vi "Kalibrationsprogramm dodenhoeft.vi"(2 "Delay [ms]":u32=10000, 3 "Messzeit [ms]":u32=7000, 4 "B-Feld":dbl=4.0, 5 "error in (no error)":errorcluster, 6 "Startwert (V)":dbl=-6.0 min=-30.0 max=30.0 step=0.01, 7 "Stepsize (V)":dbl=1.0 min=0.0, 8 "Endwert (V)":dbl=6.0 min=-30.0 max=30.0 step=0.01) -> (15 "Ausgabe-Cluster":T1={" I (A)"=-6.000000000000021, "Voltage"=0.143902, "B-Feld"=4.0, "Timestamp"=3443775799.1979947} {"Timestamp" format="%#_6f"}, 19 "error out":errorcluster)   [LabVIEW 2009]
uses:
  Instance           2 16Saved   Yokogawa .vi
  <vilib>/Utility/file.llb/Write To Spreadsheet File (DBL).vi
panel:
  out "XY Graph":cluster{dbl[], dbl[]}(graph)={[-6.000000000000005, -4.990000000000027, -3.9901000000000244, -2.9900990000000083, -1.9999999999999865, -0.9900000000000079, 2.400857290751901e-15, 1.000000000000001, 2.0000000000000018, 3.0099999999999802, 4.009899999999982, 5.009900999999998, 6.00000000000002, 4.990000000000042, 3.9901000000000395, 2.999999999999979, 1.9900000000000007, 0.9999999999999987, -1.5439038936193583e-15, -1.0000000000000018, -2.0000000000000027, -3.009999999999981, -4.009899999999983, -5.009900999999999, -6.000000000000021], [0.1439003448275862, 0.14384071428571427, 0.14379167857142858, 0.14374593103448274, 0.14371203448275863, 0.14368321428571423, 0.1436658620689656, 0.1436561034482759, 0.14365485714285722, 0.14366034482758627, 0.14367178571428574, 0.1436978571428571, 0.14372814285714283, 0.14369535714285714, 0.1436752857142857, 0.14366071428571434, 0.14365396428571436, 0.14365448275862072, 0.14366448275862076, 0.14368586206896547, 0.1437107142857143, 0.14374785714285715, 0.14379375862068966, 0.1438423214285714, 0.1439047142857143]}
  in  "file path (dialog if empty)":path=path "D:/UserData/Matthias/Messungen/MgOZnO/130215/130215_259a_kalib4T_1.txt"
  out "Done":bool=TRUE
  out "Data":bool
  out "UI":dbl=-6.000000000000021
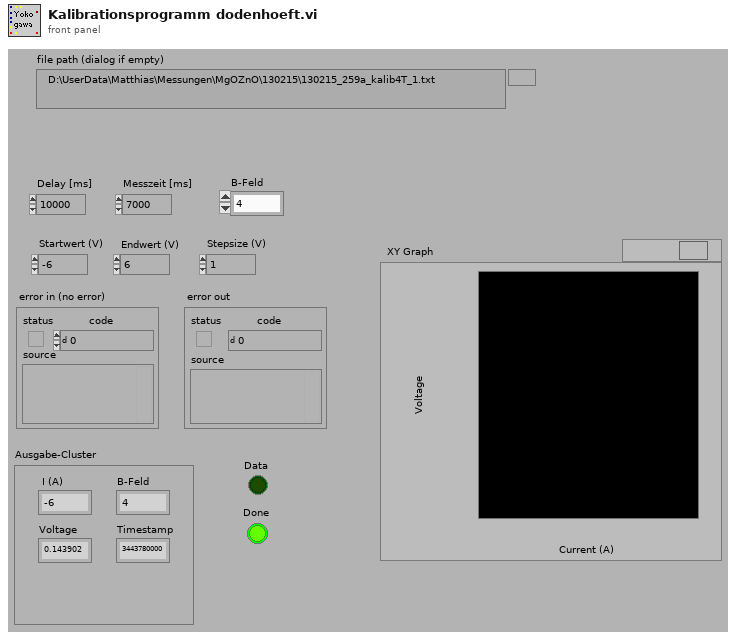
[diagram p1: front panel]
types:
  T1 = cluster{" I (A)":dbl, "Voltage":dbl, "B-Feld":dbl, "Timestamp":dbl}
  T2 = cluster{"UI":dbl, "capacitance":dbl, "B-Feld":dbl, dbl}
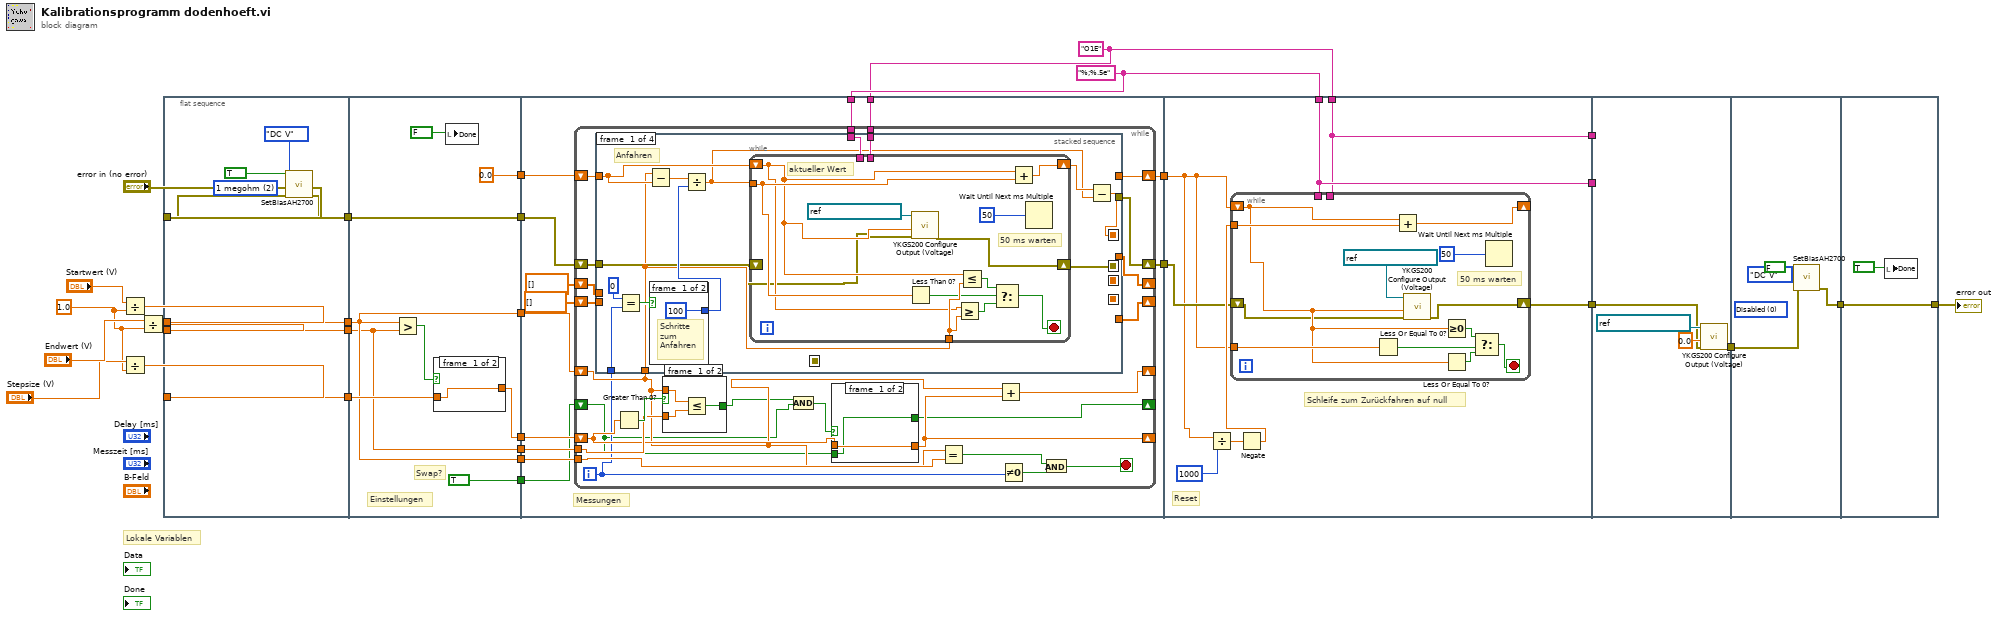
[diagram p0: block diagram]
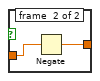
[diagram p2: hidden frame]
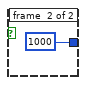
[diagram p3: hidden frame]
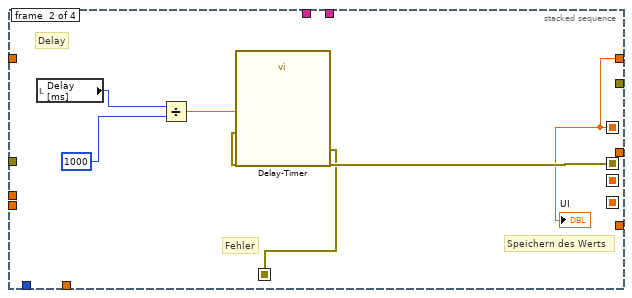
[diagram p4: hidden frame]
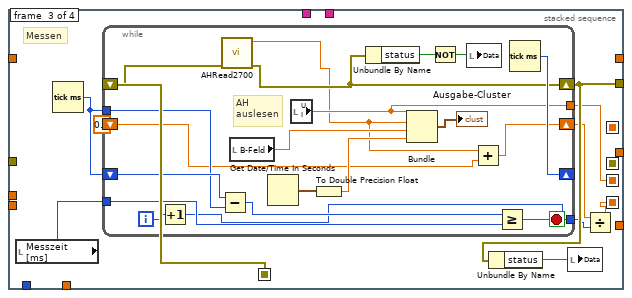
[diagram p5: hidden frame]
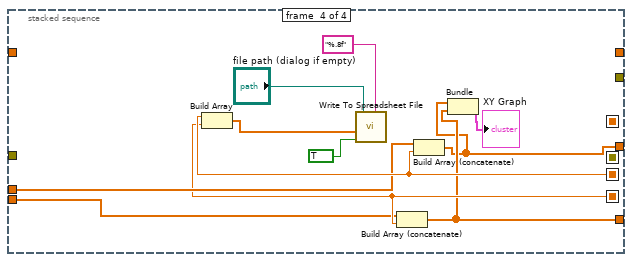
[diagram p6: hidden frame]
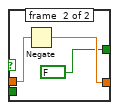
[diagram p7: hidden frame]
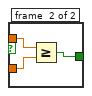
[diagram p8: hidden frame]
diagram:
  w7 = 1.0 ("y")
  w19 = "O1E"
  w20 = "%;%.5e"
  # "Lokale Variablen"
  n1 = Divide(x="Startwert (V)", y=w7) -> (x/y=w12:dbl)
  n2 = Divide(x="Stepsize (V)", y=w7) -> (x/y=w8:dbl)
  n3 = Divide(x="Endwert (V)", y=w7) -> (x/y=w10:dbl)
  n4 = flat-sequence {
    tunnel: "error in (no error)" -> [w33]
    tunnel: w8 -> [w35]
    tunnel: w10 -> [w36]
    tunnel: w12 -> [w37]
    tunnel: [w37] -> w6
    tunnel: [w36] -> w5
    tunnel: [w35] -> w4
    tunnel: [w32] -> w3
    tunnel: [w43] -> w29
    tunnel: [w44] -> w28
    tunnel: [w43] -> w27
    tunnel: [w42] -> w26
    tunnel: [0.0] -> w25
    tunnel: [w38] -> w24
    tunnel: [TRUE] -> w23
    tunnel: w6 -> [w43]
    tunnel: w5 -> [w42]
    tunnel: w4 -> [w45]
    tunnel: w3 -> [w38]
    tunnel: w29 -> [w62]
    tunnel: w28 -> [w60]
    tunnel: w27 -> [w61]
    tunnel: w26 -> [w59]
    tunnel: w25 -> [w58]
    tunnel: w20 -> [w57]
    tunnel: w19 -> [w56]
    tunnel: w24 -> [w55]
    tunnel: w23 -> [w53]
    tunnel: [w54] -> w22
    tunnel: [w52] -> w21
    tunnel: w22 -> [w178]
    tunnel: w21 -> [w176]
    tunnel: w20 -> [w175]
    tunnel: w19 -> [w174]
    tunnel: [w177] -> w17
    tunnel: [w175] -> w15
    tunnel: [w174] -> w14
    tunnel: w17 -> [w195]
    tunnel: w15 -> [_]
    tunnel: w14 -> [_]
    tunnel: [w194] -> w1
    tunnel: [w201] -> w2
    tunnel: w1 -> [w198]
    tunnel: [w203] -> w18
    tunnel: w2 -> [w203]
    frame #0 {
      w30 = 2 items=["Disabled", "100 megohm", "1 megohm"] ("Bias (Off)")
      n5 = call "SetBiasAH2700.vi"("error in (no error)"=w33, "Bias (Off)"=w30, "V/A ?"=enum16{"DC V", "DC A"}."DC V", "On/Off"=TRUE) -> ("error out"=w32:errorcluster)  [unwired: 7 in]
    }
    frame #1 {
      # "Einstellungen"
      # "Swap?"
      n6 = Greater?(x=w43, y=w42) -> (0:w46:bool)
      n7 = case shown="False" w46 {
        tunnel: w45 -> [w47 w49]
        tunnel: [w47 w48] -> w44
        frame #0 {
        }
        frame #1 {
          n8 = Negate(x=w49) -> (-x=w48:dbl)
        }
      }
      n9 = local write "Done"(FALSE) -> ()
    }
    frame #2 {
      # "Messungen"
      n10 = while {
        shift-right: [w76] -> _
        shift-left: w62 -> [w78]
        tunnel: w61 -> [w87]
        shift-right: [w77] -> _
        shift-left: w60 -> [w84]
        tunnel: w59 -> [w85]
        shift-right: [w79] -> w52
        shift-left: w58 -> [w83]
        tunnel: w57 -> [w82]
        tunnel: w56 -> [w81]
        shift-right: [w75] -> w54
        shift-left: w55 -> [w80]
        shift-right: [w70] -> _
        shift-left: w53 -> [w68]
        shift-right: [w65] -> _
        shift-left: dbl[] [] -> [w66]
        shift-right: [w64] -> _
        shift-left: dbl[] [] -> [w63]
        i -> [w74]
        stop <- w71 stop-if-true
        n11 = stacked-sequence {
          seq-local: [w93 _ _ _] -> [_ w121 _ _]
          seq-local: [_ w120 _ _] -> [_ _ w129 _]
          seq-local: [w88 _ _ _] -> [_ w116 _ _]
          seq-local: [_ _ w125 _] -> [_ _ _ w158]
          seq-local: [_ _ w122 _] -> [_ _ _ w156]
          tunnel: w74 -> [w100 _ _ _]
          tunnel: w83 -> [w92 _ _ _]
          tunnel: w78 -> [w91 _ _ _]
          tunnel: w82 -> [w96 _ _ _]
          tunnel: w81 -> [w95 _ _ _]
          tunnel: w80 -> [w94 _ _ _]
          tunnel: [_ w116 _ _] -> w79
          tunnel: [_ _ w128 _] -> w75
          tunnel: w66 -> [_ _ _ w157]
          tunnel: [_ _ _ w153] -> w65
          tunnel: [_ _ _ w154] -> w64
          tunnel: w63 -> [_ _ _ w155]
          frame #0 {
            # "Anfahren"
            n12 = Equal?(x=0, y=w100) -> (x = y?=w101:bool)
            n13 = Subtract(x=w91, y=w92) -> (x-y=w98:dbl)
            n14 = case shown="True" w101 {
              tunnel: [100 1000] -> w97
              frame #0 {
                # "Schritte\nzum\nAnfahren"
              }
              frame #1 {
              }
            }
            n15 = Divide(x=w98, y=w97) -> (x/y=w89:dbl)
            n16 = while {
              shift-right: [w113] -> w90
              shift-left: w92 -> [w105]
              tunnel: w91 -> [w110]
              tunnel: w89 -> [w111]
              tunnel: w96 -> [_]
              tunnel: w95 -> [_]
              shift-right: [w102] -> w93
              shift-left: w94 -> [w104]
              stop <- w106 stop-if-true
              # "50 ms warten"
              # "aktueller Wert"
              n17 = Less Than 0?(x=w111) -> (x < 0?=w109:bool)
              n18 = call <instrlib>:"YKGS200 Configure Output (Voltage).vi"("error in (no error)"=w104, "Voltage Level (0.0 V)"=w105, "VISA resource name"=refnum<visa-resource-name> "GPIB0::6::INSTR") -> ("error out"=w102:errorcluster)  [unwired: 7 in, 1 out]
              n19 = Greater Or Equal?(x=w105, y=w110) -> (x >= y?=w107:bool)
              n20 = Less Or Equal?(x=w105, y=w110) -> (x <= y?=w108:bool)
              n21 = Select(t=w108, s=w109, f=w107) -> (s? t:f=w106:bool)
              n22 = Add(x=w105, y=w111) -> (x+y=w113:dbl)
              n23 = Wait Until Next ms Multiple(millisecond multiple=50) -> ()  [unwired: 1 out]
            }
            n24 = Subtract(x=w90, y=w89) -> (x-y=w88:dbl)
          }
          frame #1 {
            # "Delay"
            # "Speichern des Werts"
            # "Fehler"
            n25 = local read "Delay [ms]"() -> (w117:u32)
            n26 = Divide(x=w117, y=u32 1000) -> (x/y=w118:dbl)
            n27 = call "Delay-Timer"("error in (no error)"=w121, "Delay Time (s)"=w118) -> ("error out"=w120:errorcluster)  [unwired: 9 in]
            "UI" <- w116
          }
          frame #2 {
            # "Messen"
            n28 = local read "Messzeit [ms]"() -> (w130:u32)
            n29 = Tick Count (ms)() -> (millisecond timer value=w131:u32)
            n30 = while {
              shift-right: [w151] -> _
              shift-left: w131 -> [w150]
              tunnel: w131 -> [w149]
              tunnel: w130 -> [w147]
              shift-right: [w133] -> w128
              shift-left: w129 -> [w134]
              shift-right: [w139] -> w124
              shift-left: 0.0 -> [w138]
              tunnel: [w137] -> w125
              tunnel: [w135] -> w123
              i -> [w136]
              stop <- w148 stop-if-true
              # "AH\nauslesen"
              n31 = Increment(x=w136) -> (x+1=w135:i32)
              n32 = Subtract(x=w150, y=w149) -> (x-y=w146:u32)
              n33 = call "AHRead2700.vi"("error in (no error)"=w134) -> ("error out"=w133:errorcluster, "capacitance"=w132:dbl)  [unwired: 8 in, 1 out]
              n34 = local read "B-Feld"() -> (w144:dbl)
              n35 = Get Date/Time In Seconds() -> (seconds since 1Jan1904=w145:timestamp)
              n36 = local read "UI"() -> (w137:dbl)
              n37 = To Double Precision Float(number=w145) -> (double precision float=w143:dbl)
              n38 = Unbundle By Name(w133) -> ("status"=w142:bool)
              n39 = Bundle("UI"=w137, "capacitance"=w132, "B-Feld"=w144, w143) -> (→"Ausgabe-Cluster":T2)  [unwired: 1 in]
              n40 = Not(x=w142) -> (.not. x?=w141:bool)
              n41 = local write "Data"(w141) -> ()
              n42 = Add(x=w132, y=w138) -> (x+y=w139:dbl)
              n43 = Greater Or Equal?(x=w146, y=w147) -> (x >= y?=w148:bool)
              n44 = Tick Count (ms)() -> (millisecond timer value=w151:u32)
            }
            n45 = Unbundle By Name(w128) -> ("status"=w127:bool)
            n46 = local write "Data"(w127) -> ()
            n47 = Divide(x=w124, y=w123) -> (x/y=w122:dbl)
          }
          frame #3 {
            n48 = Build Array(w158, w156) -> (w162:dbl[])
            n49 = call-poly <vilib>:"Write To Spreadsheet File.vi"("format (%.3f)"="%.8f", "append to file? (new file:F)"=TRUE, "1D data"=w162, "file path (dialog if empty)"="file path (dialog if empty)") -> ()  [unwired: 4 in, 1 out]
            n50 = Build Array (concatenate)(w155, w156) -> (w154:dbl[])
            n51 = Build Array (concatenate)(w157, w158) -> (w153:dbl[])
            n52 = Bundle(w153, w154) -> (→"XY Graph":cluster{dbl[], dbl[]})  [unwired: 1 in]
          }
        }
        n53 = Greater Than 0?(x=w84) -> (x > 0?=w86:bool)
        n54 = case shown="True" w86 {
          tunnel: w85 -> [w169 w172]
          tunnel: w78 -> [w170 w173]
          tunnel: [w168 w171] -> w69
          frame #0 {
            n55 = Less Or Equal?(x=w170, y=w169) -> (x <= y?=w168:bool)
          }
          frame #1 {
            n56 = Greater Or Equal?(x=w173, y=w172) -> (x >= y?=w171:bool)
          }
        }
        n57 = And(x=w69, y=w68) -> (x .and. y?=w67:bool)
        n58 = case shown="False" w67 {
          tunnel: w84 -> [w164 w167]
          tunnel: [w164 w166] -> w77
          tunnel: [w163 FALSE] -> w70
          tunnel: w68 -> [w163 _]
          frame #0 {
          }
          frame #1 {
            n59 = Negate(x=w167) -> (-x=w166:dbl)
          }
        }
        n60 = Equal?(x=w78, y=w87) -> (x = y?=w73:bool)
        n61 = Add(x=w78, y=w77) -> (x+y=w76:dbl)
        n62 = Not Equal To 0?(x=w74) -> (x != 0?=w72:bool)
        n63 = And(x=w73, y=w72) -> (x .and. y?=w71:bool)
      }
    }
    frame #3 {
      # "Schleife zum Zurückfahren auf null"
      # "Reset"
      n64 = Divide(x=w176, y=1000) -> (x/y=w180:dbl)
      n65 = Negate(x=w180) -> (-x=w179:dbl)
      n66 = while {
        shift-right: [w188] -> _
        shift-left: w176 -> [w184]
        tunnel: w179 -> [w192]
        tunnel: w175 -> [_]
        tunnel: w174 -> [_]
        shift-right: [w182] -> w177
        shift-left: w178 -> [w183]
        tunnel: w176 -> [w187]
        stop <- w186 stop-if-true
        # "50 ms warten"
        n67 = Less Or Equal To 0?(x=w187) -> (x <= 0?=w191:bool)
        n68 = Add(x=w184, y=w192) -> (x+y=w188:dbl)
        n69 = call <instrlib>:"YKGS200 Configure Output (Voltage).vi"("error in (no error)"=w183, "Voltage Level (0.0 V)"=w184, "VISA resource name"=refnum<visa-resource-name> "GPIB0::6::INSTR") -> ("error out"=w182:errorcluster)  [unwired: 7 in, 1 out]
        n70 = Greater Or Equal To 0?(x=w184) -> (x >= 0?=w190:bool)
        n71 = Less Or Equal To 0?(x=w184) -> (x <= 0?=w189:bool)
        n72 = Select(t=w190, s=w191, f=w189) -> (s? t:f=w186:bool)
        n73 = Wait Until Next ms Multiple(millisecond multiple=50) -> ()  [unwired: 1 out]
      }
    }
    frame #4 {
      n74 = call <instrlib>:"YKGS200 Configure Output (Voltage).vi"("error in (no error)"=w195, "Voltage Level (0.0 V)"=0.0, "VISA resource name"=refnum<visa-resource-name> "GPIB0::6::INSTR") -> ("error out"=w194:errorcluster)  [unwired: 7 in, 1 out]
    }
    frame #5 {
      (unwired) 0 items=["Disabled", "100 megohm", "1 megohm"] ("Bias (Off)")
      n75 = call "SetBiasAH2700.vi"("error in (no error)"=w198, "V/A ?"=enum16{"DC V", "DC A"}."DC V", "On/Off"=FALSE) -> ("error out"=w201:errorcluster)  [unwired: 8 in]
    }
    frame #6 {
      n76 = local write "Done"(TRUE) -> ()
    }
  }
  "error out" <- w18
